vi "Zählerwerte_lesen_FGV.vi"(0 "Band/Station Index":T2, 2 "gesammelte Zählerwerte":u16[](array[numeric]), 4 "Modus":T1(ring)) -> (5 "Zählerwert 1":u16, 6 "Zählerwert 2":u16, 7 "Zählerwert 3":u16)   [LabVIEW 2013, in "cRIO_FPGA_COMMUNICATION.lvlib"]
uses:
  TYPES/TYPE Station Index.ctl
  cRIO_FPGA_COMMUNICATION.lvlib
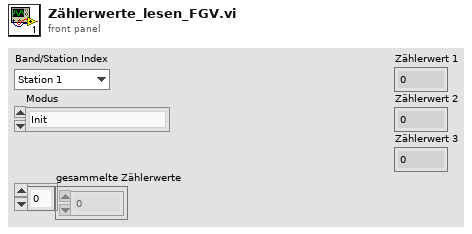
[diagram p1: front panel]
types:
  T1 = enum16{"Init", "Zählerwert updaten", "Zählerwert lesen"}
  T2 = typedef "cRIO_FPGA_COMMUNICATION.lvlib/TYPE Station Index.ctl" = enum16{"Station 1", "Station 2", "Station 3", "Station 4", "Station 5", "Station 6", "Station 7", "Station 8", "Station 9", "Station 10", "Station 11", "Station 12", "Station 13", "Station 14", "Station 15", "Station 16", "Station 17", "Station 18", "Station 19", "Station 20"}
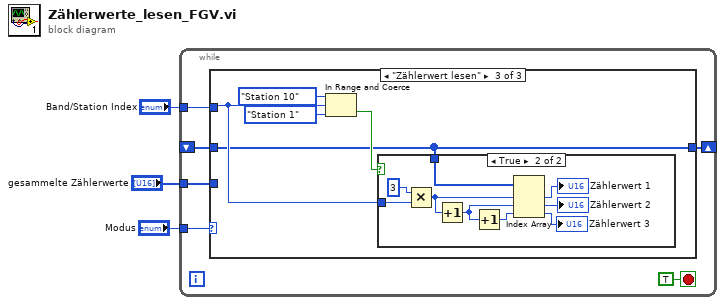
[diagram p0: block diagram]
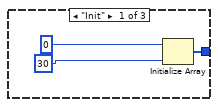
[diagram p2: hidden frame]
diagram:
  n1 = while {
    tunnel: "Modus" -> [w8]
    tunnel: "Band/Station Index" -> [w7]
    shift-right: [w6] -> _
    shift-left: _ -> [w5]
    tunnel: "gesammelte Zählerwerte" -> [w4]
    stop <- TRUE stop-if-true
    n2 = case shown="\"Zählerwert lesen\"" w8 {
      tunnel: w7 -> [_ _ w15]
      tunnel: [w11 w13 w14] -> w6
      tunnel: w5 -> [_ _ w14]
      tunnel: w4 -> [_ w13 _]
      frame "Init" {
        n3 = Initialize Array(u16 0 ("Dimension"), 30 ("Dimension")) -> (w11:u16[])
      }
      frame "Zählerwert updaten" {
      }
      frame "Zählerwert lesen" {
        n4 = In Range and Coerce(upper limit=TYPE_Station_Index."Station 10" ("Obergrenze"), x=w15, lower limit=TYPE_Station_Index."Station 1" ("Untergrenze")) -> (In Range?=w16:bool)  [unwired: 1 out]
        n5 = case shown="True" w16 {
          tunnel: w15 -> [_ w26]
          tunnel: w14 -> [_ w25]
          frame False {
          }
          frame True {
            n6 = Multiply(x=3, y=w26) -> (x*y=w24:i32)
            n7 = Increment(x=w24) -> (x+1=w23:i32)
            n8 = Increment(x=w23) -> (x+1=w22:i32)
            n9 = Index Array(array=w25, index #1=w24, index #2=w23, index #3=w22) -> (element #1=→"Zählerwert 1":u16, element #2=→"Zählerwert 2":u16, element #3=→"Zählerwert 3":u16)
          }
        }
      }
    }
  }
